vi "Logger.Variant.ReadAll.Old.vi"(8 "error in (no error)":errorcluster, 11 "FilePath":path) -> (0 "error out":errorcluster, 1 "Orders":cluster{string, string, string, string}[](array[cluster]), 2 "OrdersDetails":T1[](array[typedef]))   [LabVIEW 2016]
uses:
  Sequence/Sequence.Code.SerialFormat.ctl
  Logger.Variant.Sets.ctl
  Station/Station.Changeover.State.vi
  Station/Station.Plate.Properties.ctl
  Drivers/V7310/LowLevel/V7310.Job.Sets.ctl
panel:
  in  "SerialFormat":T4
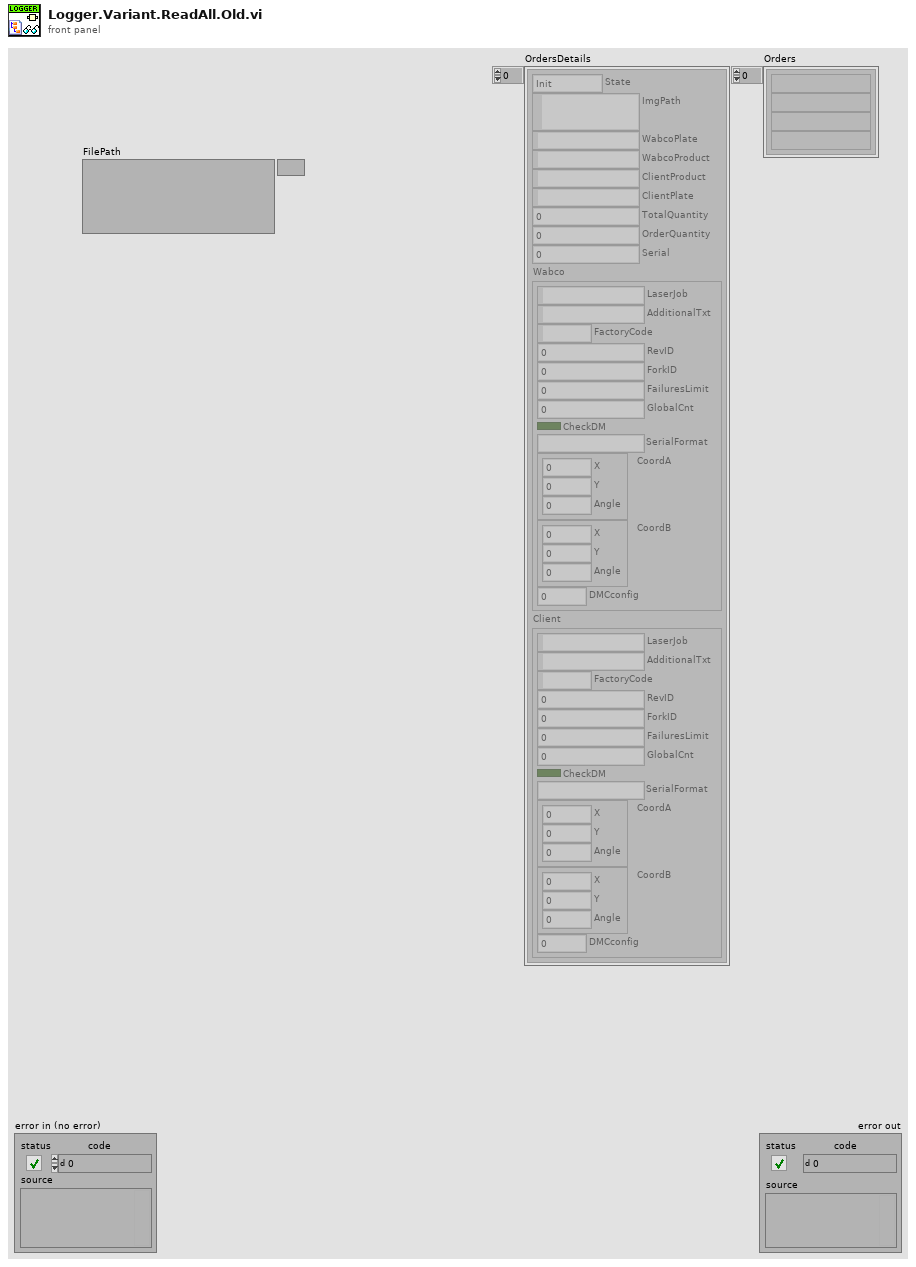
[diagram p1: front panel]
types:
  T1 = typedef "Logger.Variant.Sets.ctl" = cluster{"State":T2, "ImgPath":path, "WabcoPlate":string, "WabcoProduct":string, "ClientProduct":string, "ClientPlate":string, "TotalQuantity":u16, "OrderQuantity":u16, "Serial":i32, "Wabco":T3, "Client":T3}
  T2 = typedef "Station.Changeover.State.vi" = enum16{"Init", "Scaning", "NOK", "Wait for ack", "Ready"}
  T3 = typedef "Station.Plate.Properties.ctl" = cluster{"LaserJob":string, "AdditionalTxt":string, "FactoryCode":string, "RevID":u8, "ForkID":u8, "FailuresLimit":u16, "GlobalCnt":i32, "CheckDM":bool, "SerialFormat":T4, "CoordA":T5, "CoordB":T5, "DMCconfig":i32}
  T4 = typedef "Sequence.Code.SerialFormat.ctl" = enum8{"", "6 dig", "7 dig"}
  T5 = typedef "V7310.Job.Sets.ctl" = cluster{"X":dbl, "Y":dbl, "Angle":dbl}
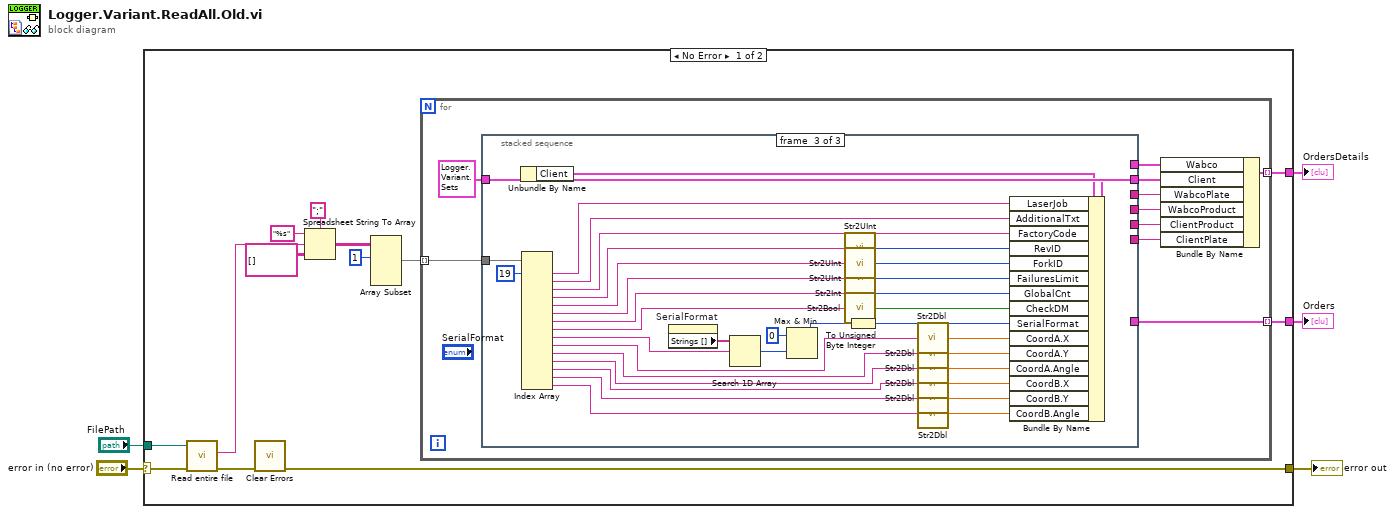
[diagram p0: block diagram]
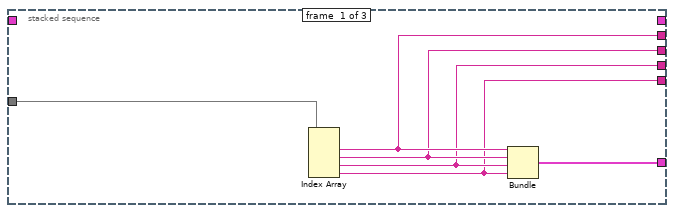
[diagram p2: hidden frame]
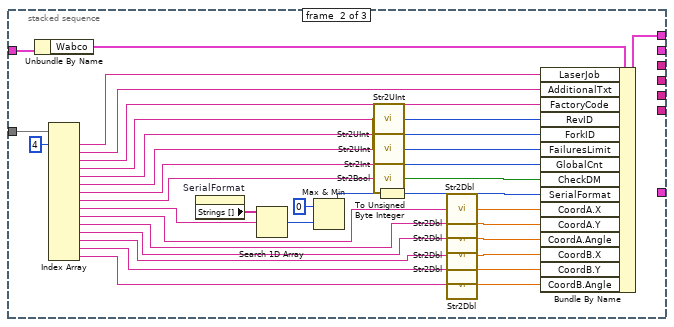
[diagram p3: hidden frame]
diagram:
  n1 = case shown="No Error" "error in (no error)" {
    selector: "error in (no error)" -> [w18 w107]
    tunnel: [w11 w107] -> w4
    tunnel: [w10 _] -> w3
    tunnel: "FilePath" -> [w7 _]
    tunnel: [w6 _] -> w1
    frame No Error {
      n2 = call "Read entire file.vi"("error in"=w18, "file"=w7) -> ("error out"=w12:errorcluster, "contents"=w17:string)  [unwired: 4 in]
      n3 = call <vilib>:"Clear Errors.vi"("error in (no error)"=w12) -> ("error out"=w11:errorcluster)  [unwired: 5 in, 1 out]
      n4 = Spreadsheet String To Array(delimiter (Tab)=";", format string="%s", spreadsheet string=w17, array type (2D Dbl)=string[][] []) -> (array=w9:string[][])
      n5 = Array Subset(array=w9, index (row)=1 ("index")) -> (w8:string[][])  [unwired: 3 in]
      n6 = for {
        tunnel: [w28] -> w10 mode=indexing
        tunnel: w8 -> [w24] mode=indexing
        tunnel: [w19] -> w6 mode=indexing
        w25 = T1 {"State"=enum."Init", "ImgPath"=path "", "WabcoPlate"="", "WabcoProduct"="", "ClientProduct"="", "ClientPlate"="", "TotalQuantity"=0, "OrderQuantity"=0, "Serial"=0, "Wabco"={"LaserJob"="", "AdditionalTxt"="037", "FactoryCode"="", "RevID"=0, "ForkID"=0, "FailuresLimit"=0, "GlobalCnt"=0, "CheckDM"=FALSE, "SerialFormat"=enum."6 dig", "CoordA"={"X"=0.0, "Y"=0.0, "Angle"=0.0}, "CoordB"={"X"=0.0, "Y"=0.0, "Angle"=0.0}, "DMCconfig"=0}, "Client"={"LaserJob"="", "AdditionalTxt"="", "FactoryCode"="037", "RevID"=0, "ForkID"=0, "FailuresLimit"=0, "GlobalCnt"=0, "CheckDM"=FALSE, "SerialFormat"=enum."6 dig", "CoordA"={"X"=0.0, "Y"=0.0, "Angle"=0.0}, "CoordB"={"X"=0.0, "Y"=0.0, "Angle"=0.0}, "DMCconfig"=0}} ("VariantSets in")
        n7 = stacked-sequence {
          tunnel: w24 -> [w34 w68 w104]
          tunnel: w25 -> [_ w38 w84]
          tunnel: [_ w66 _] -> w27
          tunnel: [_ _ w85] -> w26
          tunnel: [w33 _ _] -> w23
          tunnel: [w32 _ _] -> w22
          tunnel: [w31 _ _] -> w21
          tunnel: [w30 _ _] -> w20
          tunnel: [w29 _ _] -> w19
          frame #0 {
            n8 = Index Array(array=w34) -> (element #1=w33:string, element #2=w32:string, element #3=w31:string, element #4=w30:string)  [unwired: 4 in]
            n9 = Bundle(w33, w32, w31, w30) -> (w29:cluster{string, string, string, string})  [unwired: 1 in]
          }
          frame #1 {
            n10 = Unbundle By Name(w38) -> ("Wabco"=w70:T3)
            n11 = Index Array(array=w68, index #1=4 ("index")) -> (element #1=w67:string, element #2=w65:string, element #3=w37:string, element #4=w63:string, element #5=w35:string, element #6=w61:string, element #7=w59:string, element #8=w57:string, element #9=w45:string, element #10=w44:string, element #11=w43:string, element #12=w42:string, element #13=w41:string, element #14=w40:string, element #15=w39:string)  [unwired: 14 in]
            n12 = property on="SerialFormat" class="Enum (strict)"() -> ("Strings []"=w56:string[])  [unwired: 2 in, 2 out]
            n13 = Search 1D Array(1D array=w56, element=w45) -> (index of element=w55:i32)  [unwired: 1 in]
            n14 = Max & Min(x=0, y=w55) -> (max(x,y)=w52:i32)  [unwired: 1 out]
            n15 = call "Str2UInt.vi"("string"=w35) -> ("Numeric"=w36:u32)
            n16 = call "Str2UInt.vi"("string"=w63) -> ("Numeric"=w64:u32)
            n17 = call "Str2UInt.vi"("string"=w61) -> ("Numeric"=w62:u32)
            n18 = call "Str2Int.vi"("string"=w59) -> ("Numeric"=w60:i32)
            n19 = call "Str2Bool.vi"("string"=w57) -> ("Boolean"=w58:bool)
            n20 = To Unsigned Byte Integer(number=w52) -> (unsigned 8bit integer=w53:u8)
            n21 = call "Str2Dbl.vi"("string"=w44) -> ("Numeric"=w51:dbl)
            n22 = call "Str2Dbl.vi"("string"=w43) -> ("Numeric"=w50:dbl)
            n23 = call "Str2Dbl.vi"("string"=w42) -> ("Numeric"=w49:dbl)
            n24 = call "Str2Dbl.vi"("string"=w41) -> ("Numeric"=w48:dbl)
            n25 = call "Str2Dbl.vi"("string"=w40) -> ("Numeric"=w47:dbl)
            n26 = call "Str2Dbl.vi"("string"=w39) -> ("Numeric"=w46:dbl)
            n27 = Bundle By Name(cluster=w70, "LaserJob"=w67, "AdditionalTxt"=w65, "FactoryCode"=w37, "RevID"=w64, "ForkID"=w36, "FailuresLimit"=w62, "GlobalCnt"=w60, "CheckDM"=w58, "SerialFormat"=w53, "CoordA.X"=w51, "CoordA.Y"=w50, "CoordA.Angle"=w49, "CoordB.X"=w48, "CoordB.Y"=w47, "CoordB.Angle"=w46) -> (w66:T3)
          }
          frame #2 {
            n28 = Unbundle By Name(w84) -> ("Client"=w106:T3)
            n29 = Index Array(array=w104, index #1=19 ("index")) -> (element #1=w103:string, element #2=w102:string, element #3=w101:string, element #4=w99:string, element #5=w98:string, element #6=w96:string, element #7=w94:string, element #8=w92:string, element #9=w86:string, element #10=w81:string, element #11=w80:string, element #12=w79:string, element #13=w82:string, element #14=w83:string, element #15=w78:string)  [unwired: 14 in]
            n30 = property on="SerialFormat" class="Enum (strict)"() -> ("Strings []"=w91:string[])  [unwired: 2 in, 2 out]
            n31 = Search 1D Array(1D array=w91, element=w86) -> (index of element=w90:i32)  [unwired: 1 in]
            n32 = Max & Min(x=0, y=w90) -> (max(x,y)=w87:i32)  [unwired: 1 out]
            n33 = call "Str2UInt.vi"("string"=w99) -> ("Numeric"=w100:u32)
            n34 = call "Str2UInt.vi"("string"=w98) -> ("Numeric"=w71:u32)
            n35 = call "Str2UInt.vi"("string"=w96) -> ("Numeric"=w97:u32)
            n36 = call "Str2Int.vi"("string"=w94) -> ("Numeric"=w95:i32)
            n37 = call "Str2Bool.vi"("string"=w92) -> ("Boolean"=w93:bool)
            n38 = To Unsigned Byte Integer(number=w87) -> (unsigned 8bit integer=w88:u8)
            n39 = call "Str2Dbl.vi"("string"=w81) -> ("Numeric"=w77:dbl)
            n40 = call "Str2Dbl.vi"("string"=w80) -> ("Numeric"=w76:dbl)
            n41 = call "Str2Dbl.vi"("string"=w79) -> ("Numeric"=w75:dbl)
            n42 = call "Str2Dbl.vi"("string"=w82) -> ("Numeric"=w74:dbl)
            n43 = call "Str2Dbl.vi"("string"=w83) -> ("Numeric"=w73:dbl)
            n44 = call "Str2Dbl.vi"("string"=w78) -> ("Numeric"=w72:dbl)
            n45 = Bundle By Name(cluster=w106, "LaserJob"=w103, "AdditionalTxt"=w102, "FactoryCode"=w101, "RevID"=w100, "ForkID"=w71, "FailuresLimit"=w97, "GlobalCnt"=w95, "CheckDM"=w93, "SerialFormat"=w88, "CoordA.X"=w77, "CoordA.Y"=w76, "CoordA.Angle"=w75, "CoordB.X"=w74, "CoordB.Y"=w73, "CoordB.Angle"=w72) -> (w85:T3)
          }
        }
        n46 = Bundle By Name(cluster=w25, "Wabco"=w27, "Client"=w26, "WabcoPlate"=w23, "WabcoProduct"=w22, "ClientProduct"=w21, "ClientPlate"=w20) -> (w28:T1)
      }
    }
    frame Error {
    }
  }
  "error out" <- w4
  "OrdersDetails" <- w3
  "Orders" <- w1
